vi "rad_Configure FPGA Properties Dialog.vi"(8 "error in (no error)":errorcluster, 11 "FPGA Properties":T1) -> (0 "error out":errorcluster, 2 "Canceled":bool, 3 "FPGA Properties Out":T1)   [LabVIEW 2013]
uses:
  TypeDefs/rad_FPGA Properties.ctl
  TypeDefs/rad_FPGA Flash Properties.ctl
  Util/FP Control/FP Control Functions.ctl
panel:
  in  "Cancel":bool
  in  "Add Item":bool
  in  "Bitfile Settings":i32[](listbox)
  in  "Done":bool
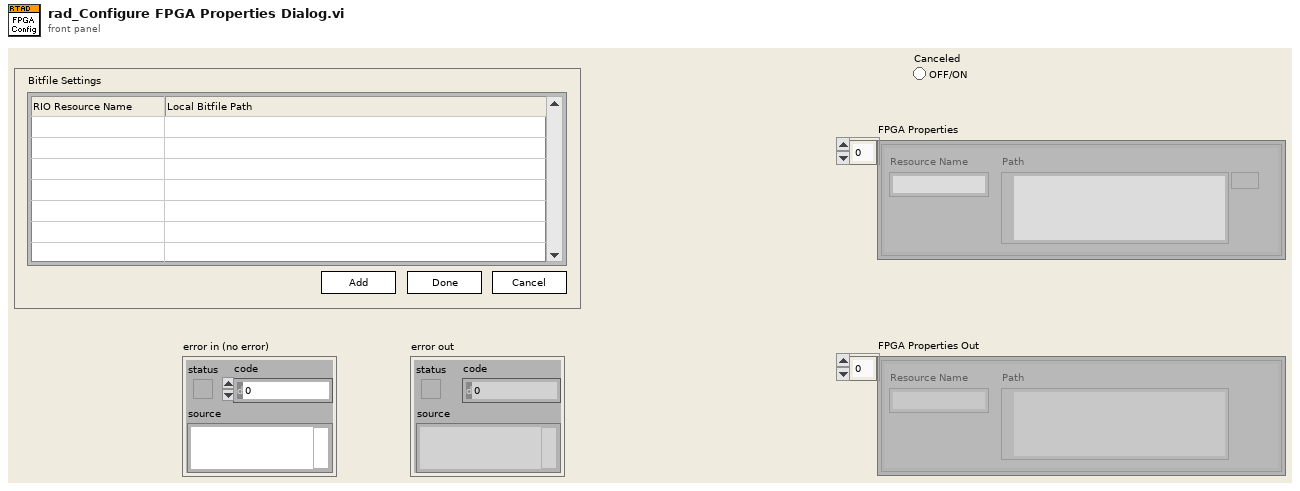
[diagram p1: front panel]
types:
  T1 = typedef "rad_FPGA Properties.ctl" = T2[]
  T2 = typedef "rad_FPGA Flash Properties.ctl" = cluster{"Resource Name":string, "Path":path}
  T3 = typedef "FP Control Functions.ctl" = enum16{"Open", "Close", "Bring To Front", "Center"}
  T4 = typedef "LVPoint32TypeDef.ctl" = cluster{"Horizontal":i32, "Vertical":i32}
  T5 = typedef "LVRowAndColumnTypeDef.ctl" = cluster{"Row":i32, "Column":i32}
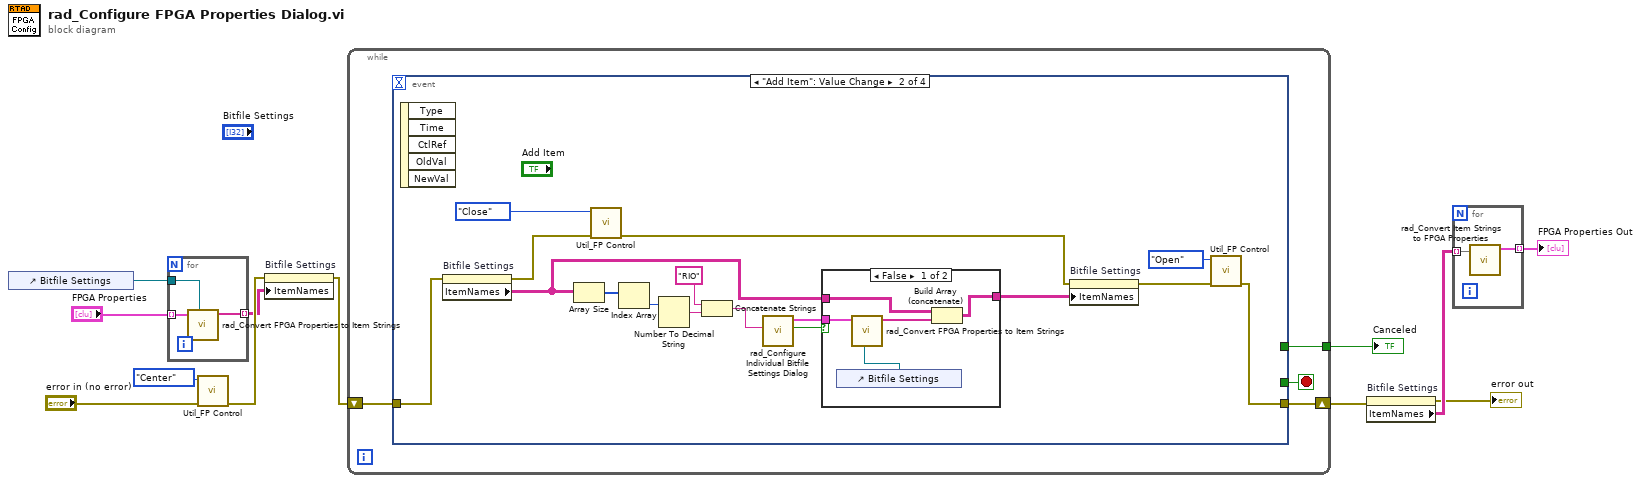
[diagram p0: block diagram]
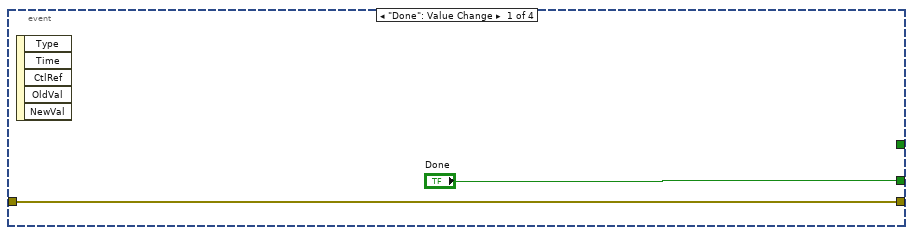
[diagram p2: hidden frame]
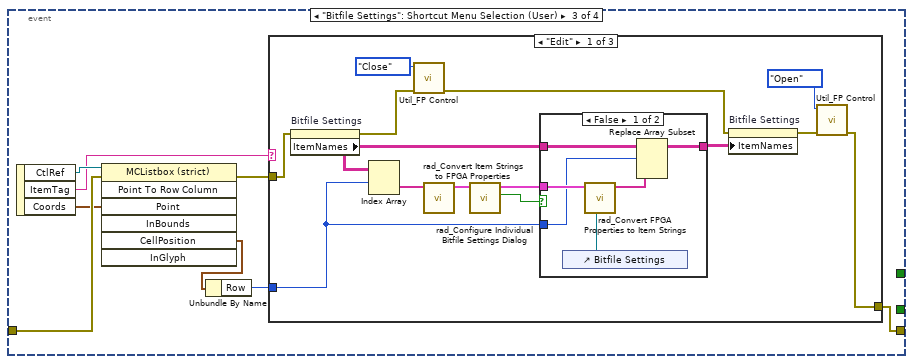
[diagram p4: hidden frame]
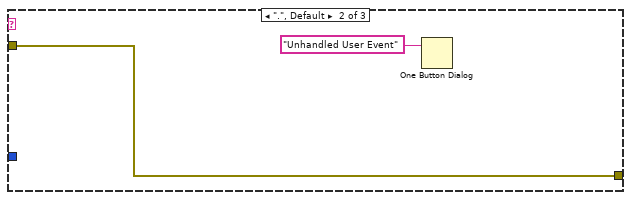
[diagram p6: hidden frame]
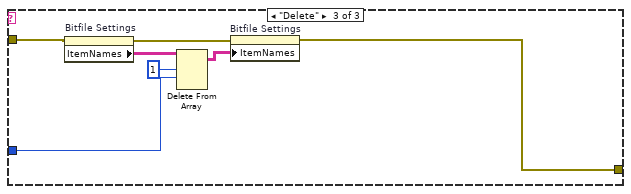
[diagram p7: hidden frame]
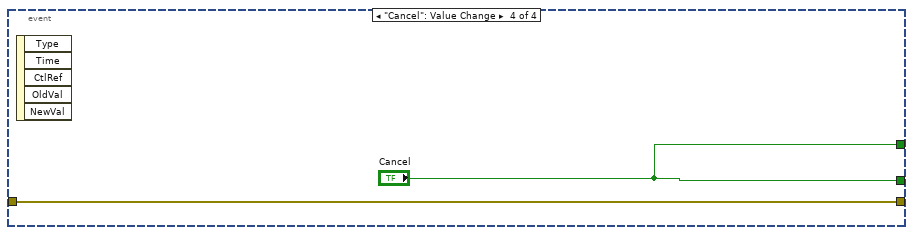
[diagram p8: hidden frame]
diagram:
  n1 = control-ref of="Bitfile Settings"() -> (w2:refnum<vi>)
  n2 = for {
    tunnel: "FPGA Properties" -> [w14] mode=indexing
    tunnel: [w15] -> w4 mode=indexing
    tunnel: w2 -> [w13]
    n3 = call "rad_Convert FPGA Properties to Item Strings.vi"("MCListbox Refnum"=w13, "FPGA Properties"=w14) -> ("Item Names"=w15:string[])  [unwired: 9 in]
  }
  n4 = call "Util_FP Control.vi"("error in (no error)"="error in (no error)", "Function"=FP_Control_Functions."Center") -> ("error out"=w6:errorcluster)  [unwired: 9 out]
  n5 = property on="Bitfile Settings" class="MCListbox (strict)"(error in=w6, "ItemNames"=w4) -> (error out=w12:errorcluster)  [unwired: 1 in, 1 out]
  n6 = while {
    tunnel: [w18] -> w11
    shift-right: [w16] -> w10
    shift-left: w12 -> [w17]
    stop <- w19 stop-if-true
    n7 = event shown="[1] \"Add Item\": Value Change" {
      selector: _ -> [_ _ _ _]
      dyn-events: _ -> [_ _ _ _]
      timeout: _ -> [_ _ _ _]
      tunnel: ["Done" _ _ "Cancel"] -> w19
      tunnel: [_ _ _ "Cancel"] -> w18
      tunnel: w17 -> [w20 w31 w50 w82]
      tunnel: [w20 w24 w44 w82] -> w16
      event "Done": Value Change {
        n8 = event-data() -> ()  [unwired: 1 in, 5 out]
      }
      event "Add Item": Value Change {
        n9 = event-data() -> ()  [unwired: 1 in, 5 out]
        n10 = property on="Bitfile Settings" class="MCListbox (strict)"(error in=w31) -> (error out=w27:errorcluster, "ItemNames"=w33:string[][])  [unwired: 1 in, 1 out]
        n11 = Array Size(array=w33) -> (size(s)=w37:i32[])
        n12 = call "Util_FP Control.vi"("error in (no error)"=w27, "Function"=FP_Control_Functions."Close") -> ("error out"=w26:errorcluster)  [unwired: 9 out]
        n13 = Index Array(array=w37) -> (element=w36:i32)  [unwired: 1 in]
        n14 = Number To Decimal String(number=w36) -> (decimal integer string=w34:string)  [unwired: 1 in]
        n15 = Concatenate Strings("RIO" ("string"), w34) -> (w23:string)
        n16 = call "rad_Configure Individual Bitfile Settings Dialog.vi"("Default RIO Resource"=w23) -> ("Canceled"=w30:bool, "FPGA Properties Out"=w22:T2)  [unwired: 8 in, 1 out]
        n17 = case shown="False" w30 {
          tunnel: w33 -> [w42 w43]
          tunnel: [w41 w43] -> w32
          tunnel: w22 -> [w40 _]
          frame False {
            n18 = control-ref of="Bitfile Settings"() -> (w38:refnum<vi>)
            n19 = call "rad_Convert FPGA Properties to Item Strings.vi"("MCListbox Refnum"=w38, "FPGA Properties"=w40) -> ("Item Names"=w39:string[])  [unwired: 9 in]
            n20 = Build Array (concatenate)(w42, w39) -> (w41:string[][])
          }
          frame True {
          }
        }
        n21 = property on="Bitfile Settings" class="MCListbox (strict)"(error in=w26, "ItemNames"=w32) -> (error out=w25:errorcluster)  [unwired: 1 in, 1 out]
        n22 = call "Util_FP Control.vi"("error in (no error)"=w25, "Function"=FP_Control_Functions."Open") -> ("error out"=w24:errorcluster)  [unwired: 9 out]
      }
      event "Bitfile Settings": Shortcut Menu Selection (User) {
        n23 = event-data() -> ("CtlRef"=w51:refnum<vi>, "ItemTag"=w45:string, "Coords"=w49:T4)  [unwired: 1 in]
        n24 = invoke class="MCListbox (strict)" method="Point To Row Column"(reference=w51, error in=w50, "Point"=w49) -> (error out=w46:errorcluster, "CellPosition"=w48:T5)  [unwired: 4 in, 5 out]
        n25 = Unbundle By Name(w48) -> ("Row"=w47:i32)
        n26 = case shown="\"Edit\"" w45 {
          tunnel: w47 -> [w55 _ w80]
          tunnel: w46 -> [w60 w73 w77]
          tunnel: [w52 w73 w75] -> w44
          frame "Edit" {
            n27 = property on="Bitfile Settings" class="MCListbox (strict)"(error in=w60) -> (error out=w61:errorcluster, "ItemNames"=w59:string[][])  [unwired: 1 in, 1 out]
            n28 = Index Array(array=w59, index (row)=w55) -> (element=w58:string[])  [unwired: 1 in]
            n29 = call "Util_FP Control.vi"("error in (no error)"=w61, "Function"=FP_Control_Functions."Close") -> ("error out"=w62:errorcluster)  [unwired: 9 out]
            n30 = call "rad_Convert Item Strings to FPGA Properties.vi"("ItemNames"=w58) -> ("FPGA Properties"=w57:T2)  [unwired: 10 in]
            n31 = call "rad_Configure Individual Bitfile Settings Dialog.vi"("FPGA Properties"=w57) -> ("Canceled"=w64:bool, "FPGA Properties Out"=w56:T2)  [unwired: 8 in, 1 out]
            n32 = case shown="False" w64 {
              tunnel: w59 -> [w69 w72]
              tunnel: [w68 w72] -> w65
              tunnel: w56 -> [w71 _]
              tunnel: w55 -> [w66 _]
              frame False {
                n33 = control-ref of="Bitfile Settings"() -> (w70:refnum<vi>)
                n34 = call "rad_Convert FPGA Properties to Item Strings.vi"("MCListbox Refnum"=w70, "FPGA Properties"=w71) -> ("Item Names"=w67:string[])  [unwired: 9 in]
                n35 = Replace Array Subset(array=w69, new element=w67, index (row)=w66) -> (w68:string[][])  [unwired: 1 in]
              }
              frame True {
              }
            }
            n36 = property on="Bitfile Settings" class="MCListbox (strict)"(error in=w62, "ItemNames"=w65) -> (error out=w53:errorcluster)  [unwired: 1 in, 1 out]
            n37 = call "Util_FP Control.vi"("error in (no error)"=w53, "Function"=FP_Control_Functions."Open") -> ("error out"=w52:errorcluster)  [unwired: 9 out]
          }
          frame ".", Default {
            n38 = One Button Dialog(message="Unhandled User Event") -> ()  [unwired: 1 in, 1 out]
          }
          frame "Delete" {
            n39 = property on="Bitfile Settings" class="MCListbox (strict)"(error in=w77) -> (error out=w76:errorcluster, "ItemNames"=w81:string[][])  [unwired: 1 in, 1 out]
            n40 = Delete From Array(array=w81, length=1, index (row)=w80) -> (array with subset deleted=w79:string[][])  [unwired: 1 in, 1 out]
            n41 = property on="Bitfile Settings" class="MCListbox (strict)"(error in=w76, "ItemNames"=w79) -> (error out=w75:errorcluster)  [unwired: 1 in, 1 out]
          }
        }
      }
      event "Cancel": Value Change {
        n42 = event-data() -> ()  [unwired: 1 in, 5 out]
      }
    }
  }
  "Canceled" <- w11
  n43 = property on="Bitfile Settings" class="MCListbox (strict)"(error in=w10) -> (error out=→"error out":errorcluster, "ItemNames"=w9:string[][])  [unwired: 1 in, 1 out]
  n44 = for {
    tunnel: w9 -> [w85] mode=indexing
    tunnel: [w84] -> w3 mode=indexing
    n45 = call "rad_Convert Item Strings to FPGA Properties.vi"("ItemNames"=w85) -> ("FPGA Properties"=w84:T2)  [unwired: 10 in]
  }
  "FPGA Properties Out" <- w3
